vi "PPS_TRAJECTORY_EXECUTE_ABS.vi"(8 "Init":bool, 11 "End Pose ENG":T7={"TRANSLATION"={"X"=0.0, "Y"=0.0}, "ROTATION"={"VALUE"=0.0, "COS"=1.0, "SIN"=0.0}} {"ROTATION"."SIN" format="%13.4f"; "ROTATION"."COS" format="%13.4f"; "ROTATION"."VALUE" format="%13.4f"; "TRANSLATION"."Y" format="%14.3f"; "TRANSLATION"."X" format="%14.3f"}) -> (0 "AtReference":bool, 3 "Chassis Velocity Target SI":T8 {"vOmega" format="%10.3f"; "vY" format="%10.3f"; "vX" format="%10.3f"})   [LabVIEW 2019]
uses:
  <vilib>/Rock Robotics/WPI/ThirdParty/JAS_Junk/TrajLib/Trajectory_Library.lvlib
  PPS_TRAJECTORY_GLOBALS.vi
  <vilib>/Rock Robotics/WPI/ThirdParty/MJansen/PathPlanner/PathPlanner24.lvlib
  <vilib>/Rock Robotics/WPI/ThirdParty/JAS_Junk/TrajLib/TypeDef/CHASSIS_SPEEDS.ctl
  <vilib>/Rock Robotics/WPI/ThirdParty/JAS_Junk/TrajLib/TypeDef/TRANSLATION2D.ctl
  <vilib>/Rock Robotics/WPI/ThirdParty/JAS_Junk/TrajLib/TypeDef/ROTATION2D.ctl
  <vilib>/Rock Robotics/WPI/ThirdParty/JAS_Junk/TrajLib/TypeDef/POSE2D.ctl
  <vilib>/Rock Robotics/WPI/ThirdParty/MJansen/PathPlanner/TypeDef/PathPlannerTrajectory.ctl
  <vilib>/Rock Robotics/WPI/ThirdParty/MJansen/PathPlanner/TypeDef/PathPlannerTrajectoryState.ctl
  <vilib>/Rock Robotics/WPI/ThirdParty/MJansen/PathPlanner/TypeDef/PathPlannerPathConstraints.ctl
panel:
  out "PathPlannerTrajectory":T1 {"States"."TargetHolonomicRotation"."SIN" format="%13.4f"; "States"."TargetHolonomicRotation"."COS" format="%13.4f"; "States"."TargetHolonomicRotation"."VALUE" format="%13.4f"; "States"."Heading"."SIN" format="%13.4f"; "States"."Heading"."COS" format="%13.4f"; "States"."Heading"."VALUE" format="%13.4f"; "States"."PositionMeters"."Y" format="%14.3f"; "States"."PositionMeters"."X" format="%14.3f"}
  in  "Robot Params":T6={"Max Module Speed M/S"=2.8, "Drive Base Radius M"=0.6}
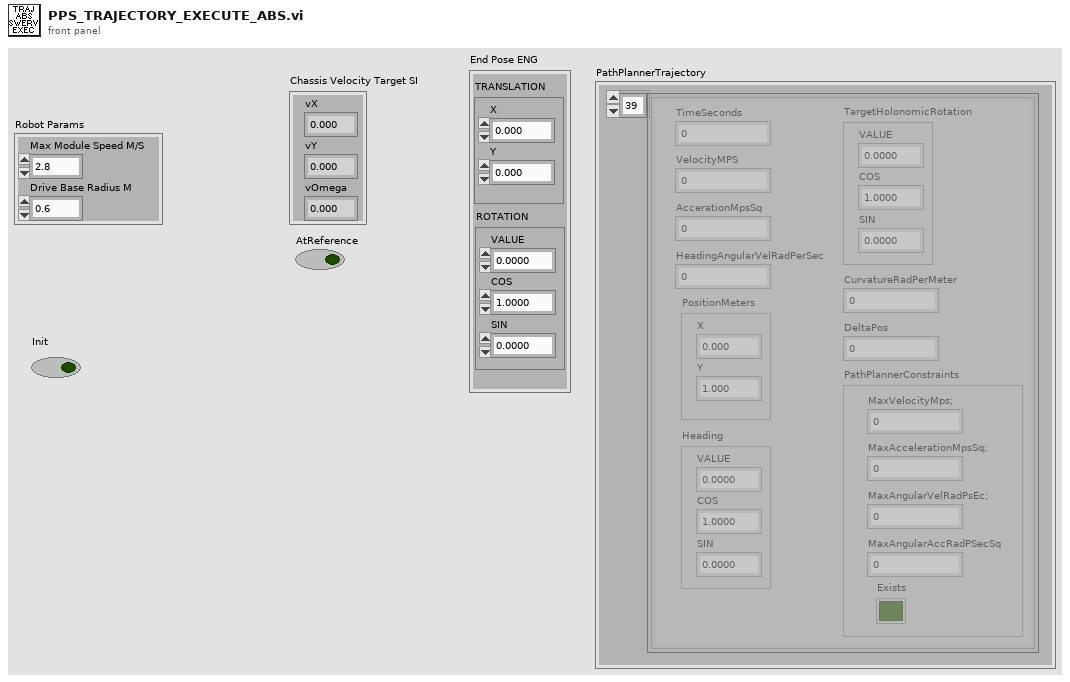
[diagram p1: front panel]
types:
  T1 = typedef "PathPlanner24.lvlib/PathPlannerTrajectory.ctl" = cluster{"States":T2[]}
  T2 = typedef "PathPlanner24.lvlib/PathPlannerTrajectoryState.ctl" = cluster{"TimeSeconds":dbl, "VelocityMPS":dbl, "AccerationMpsSq":dbl, "HeadingAngularVelRadPerSec":dbl, "PositionMeters":T3, "Heading":T4, "TargetHolonomicRotation":T4, "CurvatureRadPerMeter":dbl, "PathPlannerConstraints":T5, "DeltaPos":dbl}
  T3 = typedef "Trajectory_Library.lvlib/TRANSLATION2D.ctl" = cluster{"X":dbl, "Y":dbl}
  T4 = typedef "Trajectory_Library.lvlib/ROTATION2D.ctl" = cluster{"VALUE":dbl, "COS":dbl, "SIN":dbl}
  T5 = typedef "PathPlanner24.lvlib/PathPlannerPathConstraints.ctl" = cluster{"MaxVelocityMps;":dbl, "MaxAccelerationMpsSq;":dbl, "MaxAngularVelRadPsEc;":dbl, "MaxAngularAccRadPSecSq":dbl, "Exists":bool}
  T6 = cluster{"Max Module Speed M/S":dbl, "Drive Base Radius M":dbl}
  T7 = typedef "Trajectory_Library.lvlib/POSE2D.ctl" = cluster{"TRANSLATION":T3, "ROTATION":T4}
  T8 = typedef "Trajectory_Library.lvlib/CHASSIS_SPEEDS.ctl" = cluster{"vX":dbl, "vY":dbl, "vOmega":dbl}
  T9 = typedef "Trajectory_Library.lvlib/SWERVE_DRIVE_KINEMATICS.ctl" = cluster{"NumModules":i32, "InverseKinematics":T10, "ForwardKinematics":T10, "Modules":T3[], "PrevCoR":T3, "SavedModuleStates":T11[]}
  T10 = typedef "NI_Matrix.lvlib/RealMatrix.ctl" = dbl[][]
  T11 = typedef "Trajectory_Library.lvlib/SWERVE_DRIVE_MODULE_STATE.ctl" = cluster{"Speed":dbl, "Angle":T4}
  T12 = typedef "Trajectory_Library.lvlib/PID_TUNING.ctl" = cluster{"Kp":dbl, "Ki":dbl, "Kd":dbl, "MaximumIntegral":dbl, "MinimumIntegral":dbl}
  T13 = typedef "Trajectory_Library.lvlib/PROFILED_PID_CONTROLLER.ctl" = cluster{"Controller":T14, "Goal":T15, "Setpoint":T15, "Constraint":T16}
  T14 = typedef "Trajectory_Library.lvlib/PID_CONTROLLER.ctl" = cluster{"Kp":dbl, "Ki":dbl, "Kd":dbl, "Period":dbl, "Max_Integral":dbl, "Min_Integral":dbl, "Max_Input":dbl, "Min_Input":dbl, "Continuous":bool, "PositionError":dbl, "VelocityError":dbl, "PrevError":dbl, "TotalError":dbl, "PositionTolerance":dbl, "VelocityTolerance":dbl, "SetPoint":dbl, "Kf":dbl, "Prev_Deriv":dbl, "Prev_Deriv 2":dbl, "DerivativeFilter":bool, "Min_Output":dbl, "Max_Output":dbl, "Prev_F_P":dbl, "Prev_F_P_2":dbl, "AntiWindupActive":bool, "Measurement":dbl}
  T15 = typedef "Trajectory_Library.lvlib/TRAPEZOID_PROFILE_STATE.ctl" = cluster{"Position":dbl, "Velocity":dbl}
  T16 = typedef "Trajectory_Library.lvlib/TRAPEZOID_PROFILE_CONSTRAINT.ctl" = cluster{"MaxVelocity":dbl, "MaxAcceleration":dbl}
  T17 = typedef "Trajectory_Library.lvlib/HOLONOMIC_PACK_TUNING.ctl" = cluster{"X PID Tuning":T12, "Y PID Tuning":T12, "thetaProfiledPID_CTRL":T13}
  T18 = typedef "Trajectory_Library.lvlib/HOLONOMIC_DRV_CTRL.ctl" = cluster{"poseTolerance":T7, "poseError":T7, "Enabled":bool, "PID_xCtrl":T14, "PID_yCtrl":T14, "PROF_PID_thetaCtrl":T13, "RotationError":T4, "FirstRun":bool}
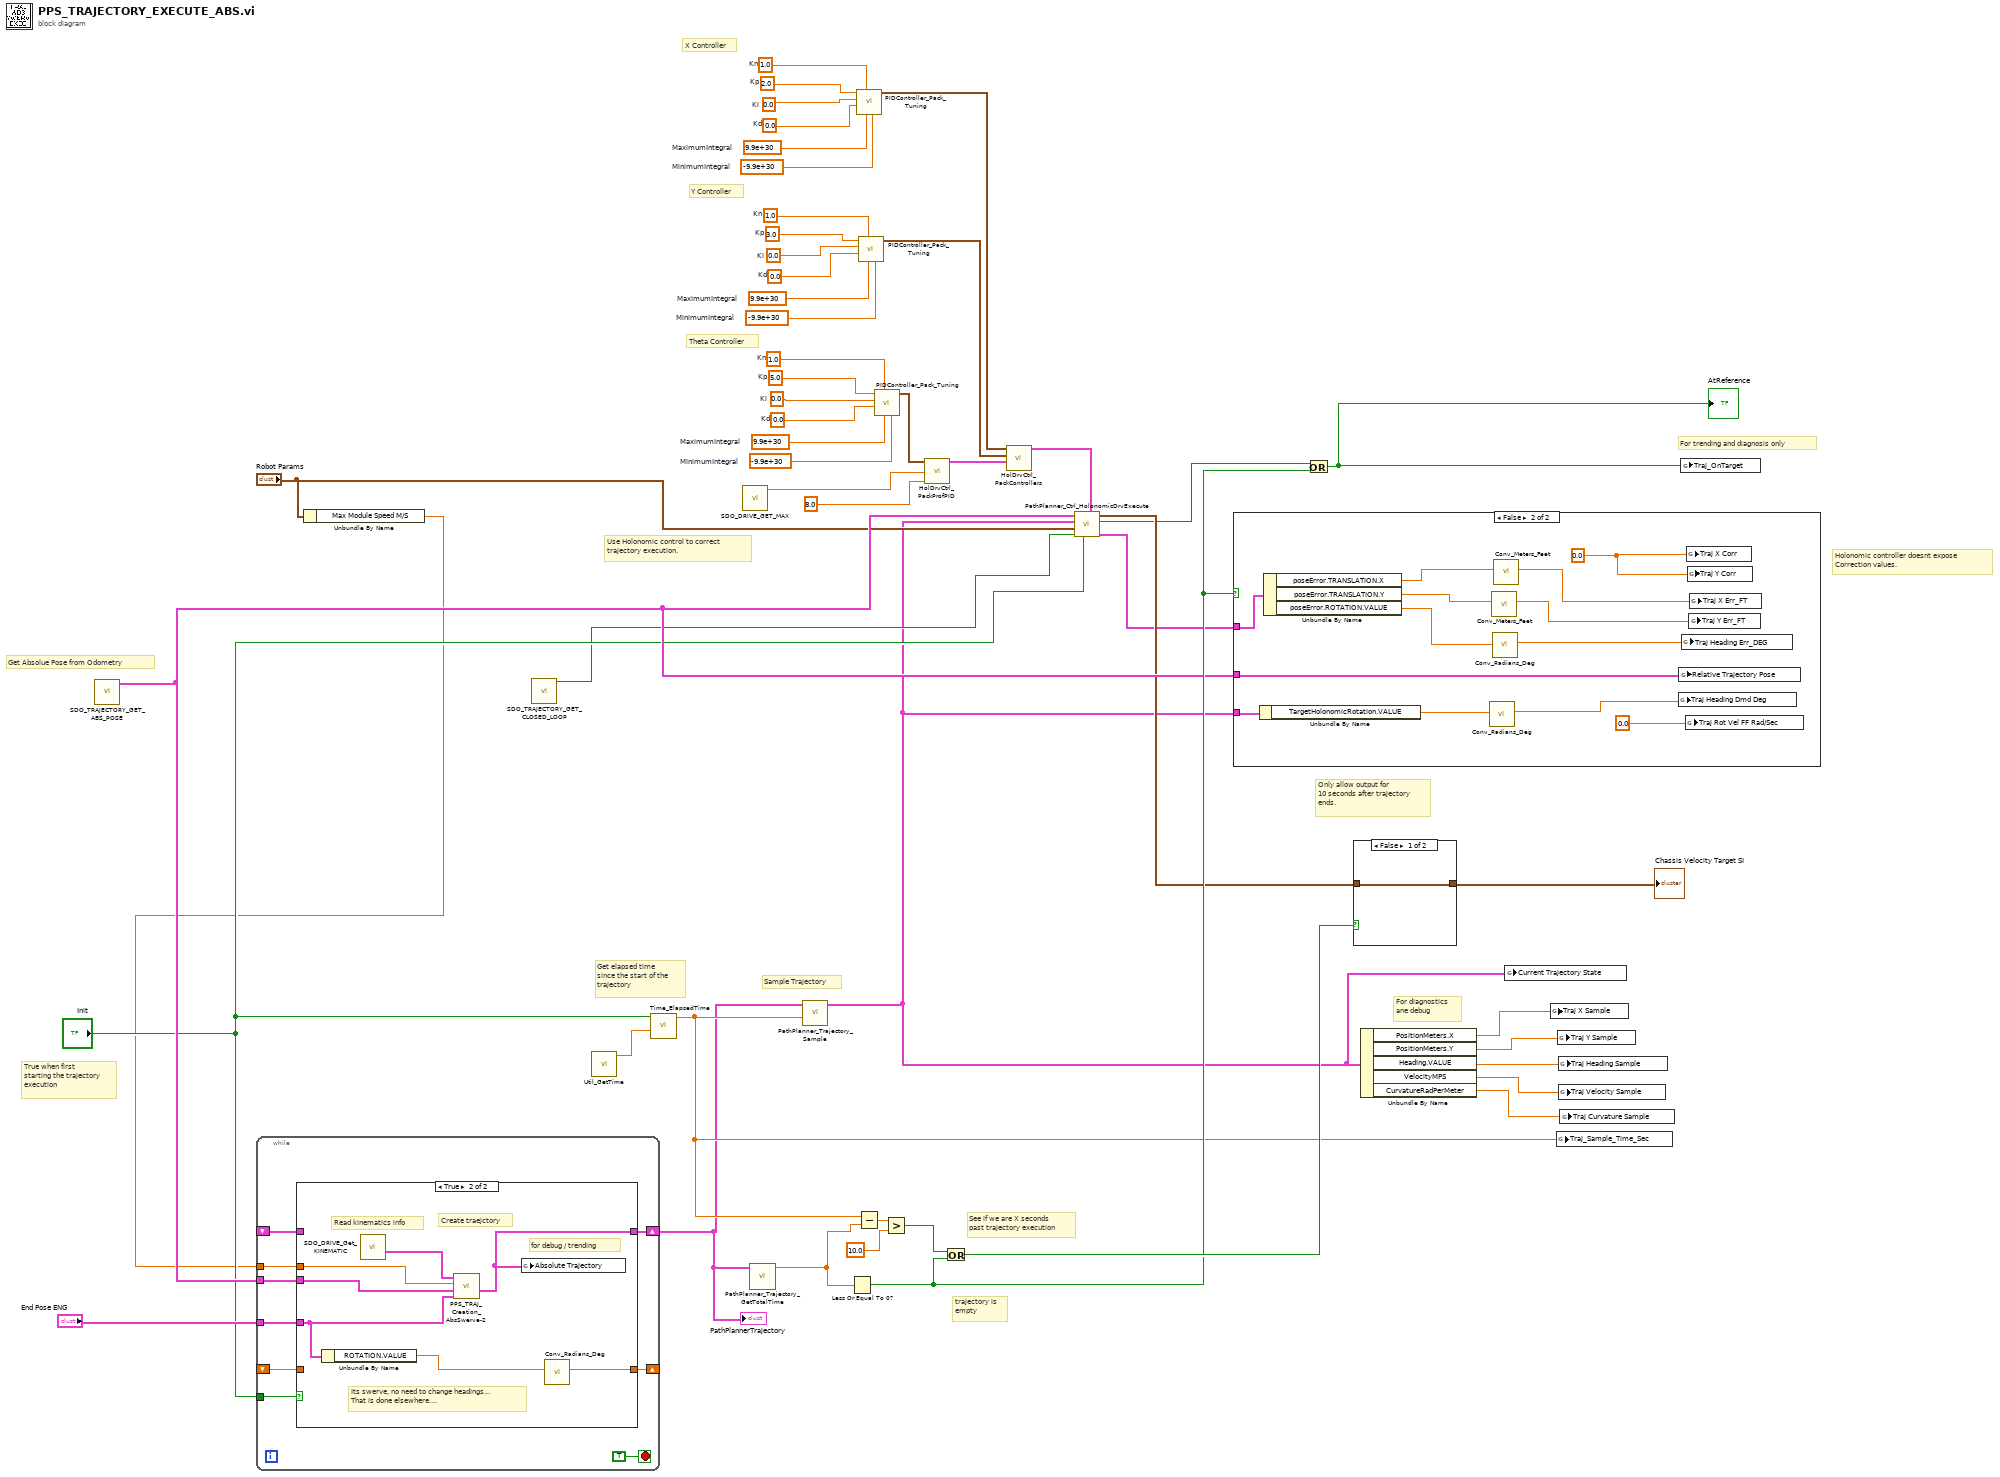
[diagram p0: block diagram]
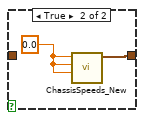
[diagram p4: hidden frame]
diagram:
  w24 = 1.0  # Kn
  w27 = 5.0  # Kp
  w36 = 0.0  # Ki
  w37 = 0.0  # Kd
  w38 = 9.9e+30  # MaximumIntegral
  w39 = -9.9e+30  # MinimumIntegral
  w22 = 1.0  # Kn
  w25 = 2.0  # Kp
  w28 = 0.0  # Ki
  w29 = 0.0  # Kd
  w30 = 9.9e+30  # MaximumIntegral
  w31 = -9.9e+30  # MinimumIntegral
  w23 = 1.0  # Kn
  w26 = 3.0  # Kp
  w32 = 0.0  # Ki
  w33 = 0.0  # Kd
  w34 = 9.9e+30  # MaximumIntegral
  w35 = -9.9e+30  # MinimumIntegral
  # "trajectory is \nempty"
  # "Theta Controller"
  # "Y Controller"
  # "X Controller"
  # "True when first\nstarting the trajectory\nexecution"
  # "Get elapsed time\nsince the start of the\ntrajectory"
  # "Holonomic controller doesnt expose\nCorrection values."
  # "Use Holonomic control to correct\ntrajectory execution."
  # "For trending and diagnosis only"
  # "For diagnostics\nane debug"
  # "Get Absolue Pose from Odometry"
  # "Sample Trajectory"
  # "See if we are X seconds \npast trajectory execution"
  # "Only allow output for\n10 seconds after trajectory\nends."
  n1 = call "SDO_TRAJECTORY_GET_ABS_POSE.vi"() -> ("Absolute Odometry Pose"=w12:T7)  [unwired: 11 in]
  n2 = Unbundle By Name("Robot Params") -> ("Max Module Speed M/S"=w4:dbl)
  n3 = while {
    tunnel: "Init" -> [w59]
    tunnel: w12 -> [w58]
    shift-right: [w57] -> w7
    shift-left: _ -> [w56]
    shift-right: [w55] -> _
    shift-left: _ -> [w54]
    tunnel: "End Pose ENG" -> [w53]
    tunnel: w4 -> [w52]
    stop <- TRUE stop-if-true
    n4 = case shown="True" w59 {
      tunnel: w58 -> [_ w64]
      tunnel: [w62 w66] -> w57
      tunnel: w56 -> [w62 _]
      tunnel: [w61 w68] -> w55
      tunnel: w54 -> [w61 _]
      tunnel: w53 -> [_ w69]
      tunnel: w52 -> [_ w63]
      frame False {
      }
      frame True {
        # "for debug / trending"
        # "Read kinematics info"
        # "Its swerve, no need to change headings...\nThat is done elsewhere...."
        # "Create traejctory"
        n5 = Unbundle By Name(w69) -> ("ROTATION.VALUE"=w67:dbl)
        n6 = call "SDO_DRIVE_Get_KINEMATIC.vi"() -> ("out SWERVE_DRIVE_KINEMATICS"=w65:T9)  [unwired: 11 in]
        n7 = call "PPS_TRAJ_Creation_AbsSwerve-2.vi"("End Pose  ENG"=w69, "Current Pose SI"=w64, "Max Velocity M/S"=w63, "SWERVE_DRIVE_KINEMATICS"=w65) -> ("PathPlannerTrajectory"=w66:T1)  [unwired: 5 in, 2 out]
        n8 = global write "PPS_TRAJECTORY_GLOBALS.vi" "Absolute Trajectory"(w66) -> ()
        n9 = call <vilib>:"Conv_Radians_Deg.vi"("Radians"=w67) -> ("Degrees"=w68:dbl)  [unwired: 10 in]
      }
    }
  }
  "PathPlannerTrajectory" <- w7
  n10 = call "SDO_TRAJECTORY_GET_CLOSED_LOOP.vi"() -> ("AUTO_CLOSED_LOOP"=w10:bool)  [unwired: 11 in]
  n11 = call <vilib>:"Util_GetTime.vi"() -> ("FPGA_Time_Seconds"=w48:dbl)  [unwired: 9 in, 2 out]
  n12 = call <vilib>:"Time_ElapsedTime.vi"("PassthroughTime_SEC"=w48, "Reset"="Init") -> ("Elapsed Time Sec"=w14:dbl)  [unwired: 9 in]
  n13 = call "SDO_DRIVE_GET_MAX.vi"() -> ("Max Wheel Vel (Meter/Sec)"=w1:dbl)  [unwired: 10 in, 1 out]
  n14 = call <vilib>:"PathPlanner_Trajectory_GetTotalTime.vi"("PathPlannerTrajectory"=w7) -> ("TotalTimeSeconds"=w6:dbl)  [unwired: 10 in]
  n15 = call <vilib>:"PathPlanner_Trajectory_Sample.vi"("Time"=w14, "PathPlannerTrajectory"=w7) -> ("PathPlannerState"=w2:T2)  [unwired: 9 in]
  n16 = Less Or Equal To 0?(x=w6) -> (x <= 0?=w15:bool)
  n17 = call <vilib>:"PIDController_Pack_Tuning.vi"("MinimumIntegral"=w31, "MaximumIntegral"=w30, "Kn"=w22, "Kd"=w29, "Ki"=w28, "Kp"=w25) -> ("PID Tuning"=w40:T12)  [unwired: 5 in]
  n18 = Subtract(x=w14, y=w6) -> (x-y=w51:dbl)
  n19 = call <vilib>:"PIDController_Pack_Tuning.vi"("MinimumIntegral"=w35, "MaximumIntegral"=w34, "Kn"=w23, "Kd"=w33, "Ki"=w32, "Kp"=w26) -> ("PID Tuning"=w41:T12)  [unwired: 5 in]
  n20 = call <vilib>:"PIDController_Pack_Tuning.vi"("MinimumIntegral"=w39, "MaximumIntegral"=w38, "Kn"=w24, "Kd"=w37, "Ki"=w36, "Kp"=w27) -> ("PID Tuning"=w21:T12)  [unwired: 5 in]
  n21 = Greater?(x=w51, y=10.0) -> (0:w18:bool)
  n22 = call <vilib>:"HolDrvCtrl_PackProfPID.vi"("Max Accel"=8.0, "Max Speed"=w1, "Theta PID Tuning"=w21) -> ("Theta PID CONTROLLER"=w42:T13)  [unwired: 8 in]
  n23 = Or(x=w18, y=w15) -> (x .or. y?=w17:bool)
  n24 = call <vilib>:"HolDrvCtrl_PackControllers.vi"("thetaProfiledPID_CTRL"=w42, "Y PID Tuning"=w41, "X PID Tuning"=w40) -> ("HOLONOMIC_CTRL_PACK_TUNING"=w13:T17)  [unwired: 8 in]
  n25 = call <vilib>:"PathPlanner_Ctrl_HolonomicDrvExecute.vi"("HOLONOMIC_CTRL_PACK_TUNING"=w13, "Reset"="Init", "Enabled"=w10, "Robot Params"="Robot Params", "PathPlannerState"=w2, "Current Pose SI"=w12) -> ("outHOLONOMIC_DRV_CTRL"=w3:T18, "At Reference"=w8:bool, "calcChassisSpeed"=w9:T8)  [unwired: 2 in, 1 out]
  n26 = case shown="False" w15 {
    tunnel: w12 -> [_ w78]
    tunnel: w3 -> [_ w76]
    tunnel: w2 -> [_ w72]
    frame True {
    }
    frame False {
      w82 = 0.0 ("Y Corr")
      n27 = Unbundle By Name(w72) -> ("TargetHolonomicRotation.VALUE"=w71:dbl)
      n28 = Unbundle By Name(w76) -> ("poseError.TRANSLATION.X"=w75:dbl, "poseError.TRANSLATION.Y"=w74:dbl, "poseError.ROTATION.VALUE"=w73:dbl)
      n29 = call <vilib>:"Conv_Radians_Deg.vi"("Radians"=w71) -> ("Degrees"=w70:dbl)  [unwired: 10 in]
      n30 = call <vilib>:"Conv_Meters_Feet.vi"("Meters"=w74) -> ("Feet"=w80:dbl)  [unwired: 10 in]
      n31 = call <vilib>:"Conv_Radians_Deg.vi"("Radians"=w73) -> ("Degrees"=w81:dbl)  [unwired: 10 in]
      n32 = call <vilib>:"Conv_Meters_Feet.vi"("Meters"=w75) -> ("Feet"=w79:dbl)  [unwired: 10 in]
      n33 = global write "PPS_TRAJECTORY_GLOBALS.vi" "Traj Heading Dmd Deg"(w70) -> ()
      n34 = global write "PPS_TRAJECTORY_GLOBALS.vi" "Relative Trajectory Pose"(w78) -> ()
      n35 = global write "PPS_TRAJECTORY_GLOBALS.vi" "Traj Heading Err_DEG"(w81) -> ()
      n36 = global write "PPS_TRAJECTORY_GLOBALS.vi" "Traj Rot Vel FF Rad/Sec"(0.0 ("Traj Heading Dmd Deg")) -> ()
      n37 = global write "PPS_TRAJECTORY_GLOBALS.vi" "Traj X Corr"(w82) -> ()
      n38 = global write "PPS_TRAJECTORY_GLOBALS.vi" "Traj Y Corr"(w82) -> ()
      n39 = global write "PPS_TRAJECTORY_GLOBALS.vi" "Traj Y Err_FT"(w80) -> ()
      n40 = global write "PPS_TRAJECTORY_GLOBALS.vi" "Traj X Err_FT"(w79) -> ()
    }
  }
  n41 = Or(x=w8, y=w15) -> (x .or. y?=w16:bool)
  "AtReference" <- w16
  n42 = case shown="False" w17 {
    tunnel: w9 -> [w83 _]
    tunnel: [w83 w84] -> w49
    frame False {
    }
    frame True {
      w85 = 0.0 ("vX")
      n43 = call <vilib>:"ChassisSpeeds_New.vi"("vAngular"=w85, "vY"=w85, "vX"=w85) -> ("CHASSIS"=w84:T8)  [unwired: 8 in]
    }
  }
  "Chassis Velocity Target SI" <- w49
  n44 = Unbundle By Name(w2) -> ("PositionMeters.X"=w47:dbl, "PositionMeters.Y"=w46:dbl, "Heading.VALUE"=w45:dbl, "VelocityMPS"=w44:dbl, "CurvatureRadPerMeter"=w43:dbl)
  n45 = global write "PPS_TRAJECTORY_GLOBALS.vi" "Current Trajectory State"(w2) -> ()
  n46 = global write "PPS_TRAJECTORY_GLOBALS.vi" "Traj X Sample"(w47) -> ()
  n47 = global write "PPS_TRAJECTORY_GLOBALS.vi" "Traj_Sample_Time_Sec"(w14) -> ()
  n48 = global write "PPS_TRAJECTORY_GLOBALS.vi" "Traj Y Sample"(w46) -> ()
  n49 = global write "PPS_TRAJECTORY_GLOBALS.vi" "Traj Heading Sample"(w45) -> ()
  n50 = global write "PPS_TRAJECTORY_GLOBALS.vi" "Traj Velocity Sample"(w44) -> ()
  n51 = global write "PPS_TRAJECTORY_GLOBALS.vi" "Traj Curvature Sample"(w43) -> ()
  n52 = global write "PPS_TRAJECTORY_GLOBALS.vi" "Traj_OnTarget"(w16) -> ()
